vi "Get Header.vi"(8 "error in (no error)":errorcluster, 10 "header":string(combo)="User-Agent", 11 "HTTP Client Base in":refnum<class "LabVIEW HTTP Client.lvclass">) -> (0 "error out":errorcluster, 2 "value":string, 3 "HTTP Client Base out":refnum<class "LabVIEW HTTP Client.lvclass">)   [LabVIEW 2021, in "HTTP Client Abstract.lvlib" / "LabVIEW HTTP Client.lvclass"]
uses:
  LabVIEW HTTP Client.lvclass
  LabVIEW HTTP Client.lvclass/LabVIEW HTTP Client.ctl
  <vilib>/httpClient/LabVIEWHTTPClient.lvlib
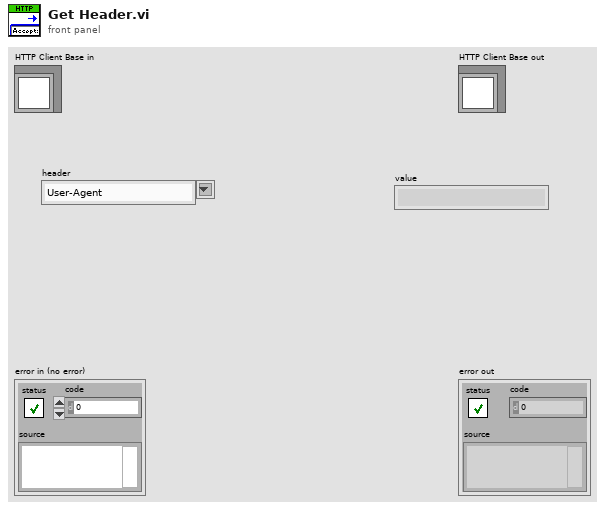
[diagram p1: front panel]
types:
  T1 = typedef "LabVIEWHTTPClient.lvlib/ClientHandle.ctl" = refnum<k1>
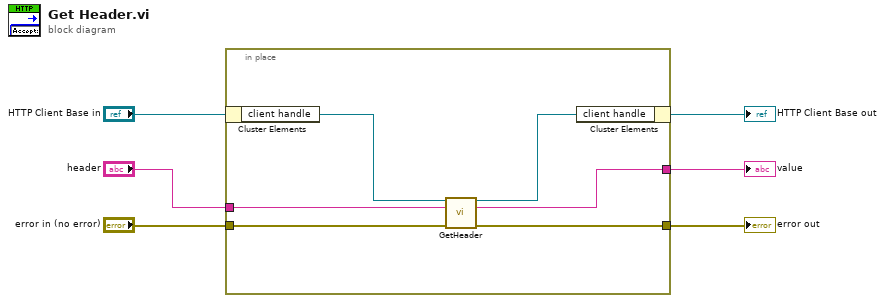
[diagram p0: block diagram]
diagram:
  n1 = in-place {
    in-place-border: "error in (no error)" -> [w12]
    in-place-border: [w11] -> w5
    in-place-border: "header" -> [w8]
    in-place-border: [w7] -> w1
    n2 = in-place-cluster #1("HTTP Client Base in") -> ("client handle"=w9:T1)
    n3 = call <vilib>:"GetHeader.vi"("client handle"=w9, "header"=w8, "error in (no error)"=w12) -> ("client handle out"=w10:T1, "value"=w7:string, "error out"=w11:errorcluster)  [unwired: 10 in]
    n4 = in-place-cluster #1("client handle"=w10) -> (→"HTTP Client Base out":refnum<class "LabVIEW HTTP Client.lvclass">)
  }
  "error out" <- w5
  "value" <- w1
